vi "Zero Axis.vi"(10 "Axis":T1, 11 "VISA resource name":refnum<visa-resource-name>) -> ()   [LabVIEW 2011]
uses:
  Public/Utility/Axis Name.ctl
  Public/Utility/Serial Response Syntax.ctl
  ASI TG-1000.lvlib
panel:
  out "Command":string
  out "Command Accepted?":bool
  out "Response":string
  out "error out":errorcluster
  # "NB: this VI opens and closes the comm port"
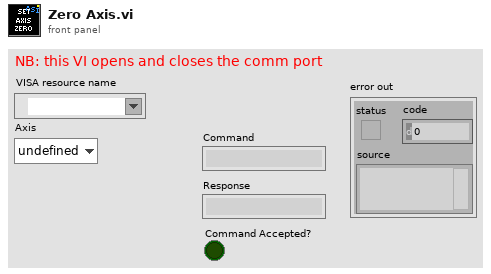
[diagram p1: front panel]
types:
  T1 = typedef "ASI TG-1000.lvlib/Axis Name.ctl" = enum8{"undefined", "A", "B", "C", "D", "E", "F", "G", "H", "I", "J", "K", "L", "M", "N", "O", "P", "Q", "R", "S", "T", "U", "V", "W", "X", "Y", "Z"}
  T2 = typedef "ASI TG-1000.lvlib/Serial Response Syntax.ctl" = enum16{":A then single line", "Single line, no :A", ":A or : then single line", ":A then single number", ":A or : then single number", ":A then <axis>= single number"}
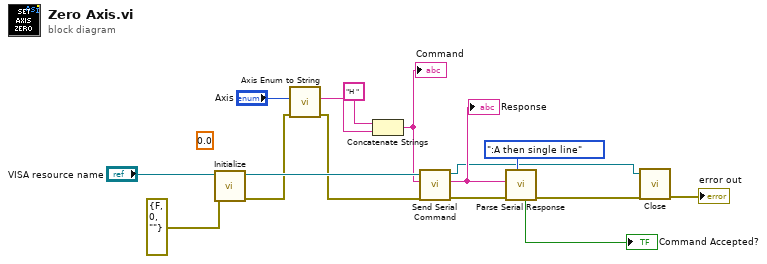
[diagram p0: block diagram]
diagram:
  (unwired) 0.0 ("Speed (mm/s)")
  n1 = call "Initialize.vi"("error in (no error)"=errorcluster {"status"=FALSE, "code"=0, "source"=""}, "VISA resource name"="VISA resource name") -> ("error out"=w10:errorcluster, "VISA resource name out"=w16:refnum<visa-resource-name>)  [unwired: 8 in]
  n2 = call "Axis Enum to String.vi"("error in (no error)"=w10, "Axis Enum In"="Axis") -> ("error out"=w9:errorcluster, "Axis String Out"=w8:string)  [unwired: 8 in]
  n3 = Concatenate Strings("H " ("Command"), w8) -> (w7:string)
  "Command" <- w7
  n4 = call "Send Serial Command.vi"("error in (no error)"=w9, "Command"=w7, "VISA in"=w16) -> ("error out"=w5:errorcluster, "Response"=w3:string, "VISA out"=w2:refnum<visa-resource-name>)  [unwired: 6 in]
  "Response" <- w3
  n5 = call "Parse Serial Response.vi"("Response Syntax"=Serial_Response_Syntax.":A then single line", "error in (no error)"=w5, "Raw Response"=w3) -> ("error out"=w4:errorcluster, "As expected?"=→"Command Accepted?":bool)  [unwired: 5 in, 2 out]
  n6 = call "Close.vi"("error in (no error)"=w4, "VISA resource name"=w2) -> ("error out"=→"error out":errorcluster)  [unwired: 9 in]
